vi "Traverse_Space_for new collision code.vi"(9 "Show Panel?":bool, 10 "Traverse Setup":string) -> (3 "Error Comments":string)   [LabVIEW 2016]
doc: "This is an example of using features of the VI Server as a client. It shows how you might browse from one or more applications that may be exporting data from one or more data stations. \n\nThe example shows how to query a server for its list of exported VIs, how to get references to the VIs, and how call them with the Call By Reference function."
uses:
  Route mapping/Box_size.ctl
  Controls/ok_button.ctl
  Collision_Detection/Triangles/EnFlo specific/Collision Detection global.vi
  Globals/Constants_global.vi
  Route mapping/Route_mapping_global.vi
panel:
  in  "Model Name":u16(ring) items=["DIPLOS_array", "Elysee", "Elysee_original", "Elysee_Source1", "Elysee_Source2", "Elysee_Source3", "MAGIC_London_Southbank_0_deg", "MAGIC_London_Southbank_0_deg_excl_12_and_150", "None", "Simple_C", "Simple_V"]
  in  "Traverse Name":u16(ring) items=["EnFlo_Stack", "EnFlo_Trav1", "EnFlo_Trav3", "EnFlo_Trav4", "EnFlo_Tunnel", "EnFlo_Turntable"]
  in  "Cancel Button":bool
  in  "OK":T1
  in  "Traverse Limits":T2=[{"Max"=15001.0, "Min"=12000.0}, {"Max"=1000.0, "Min"=-1000.0}, {"Max"=700.0, "Min"=0.0}] {"Min" format="%#.1f"; "Max" format="%#.1f"}
  # "Enter all coordinates assuming the Model Orientation is zero degrees"
  # "X                           Y                          Z"
  # "All geometry always reloaded after running this panel"
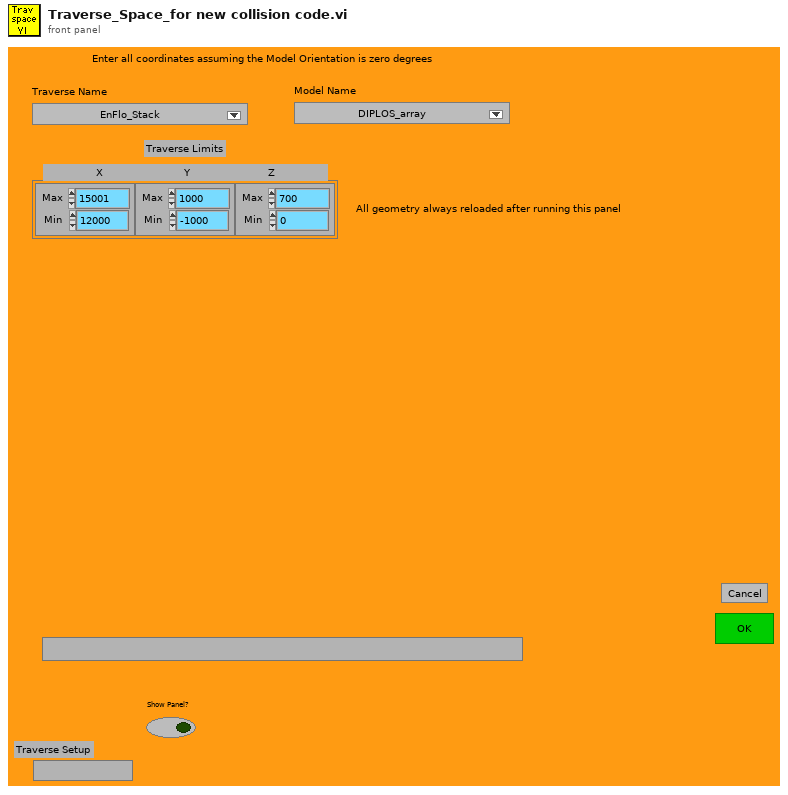
[diagram p1: front panel]
types:
  T1 = typedef "ok_button.ctl" = bool
  T2 = typedef "Box_size.ctl" = cluster{"Max":sgl, "Min":sgl}[]
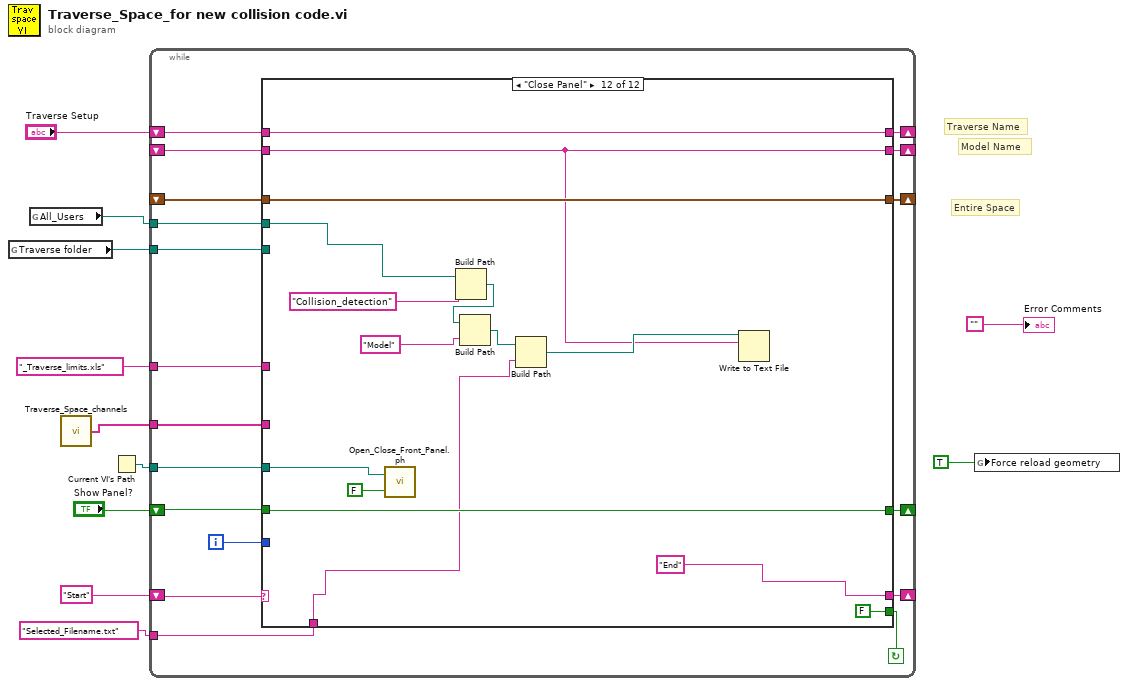
[diagram p0: block diagram]
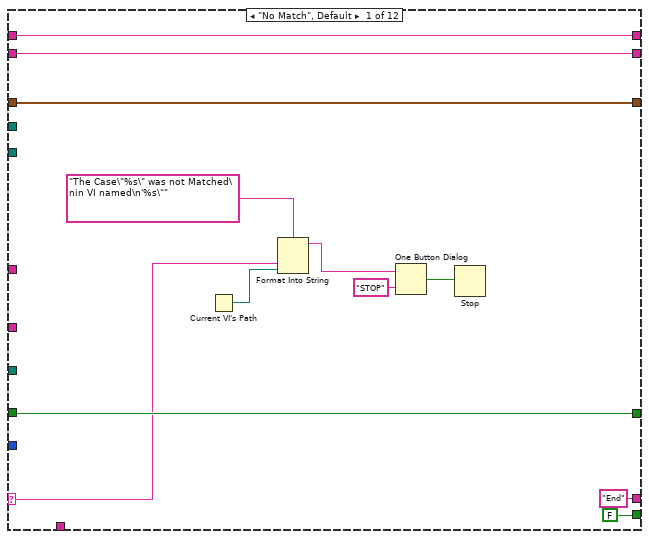
[diagram p2: hidden frame]
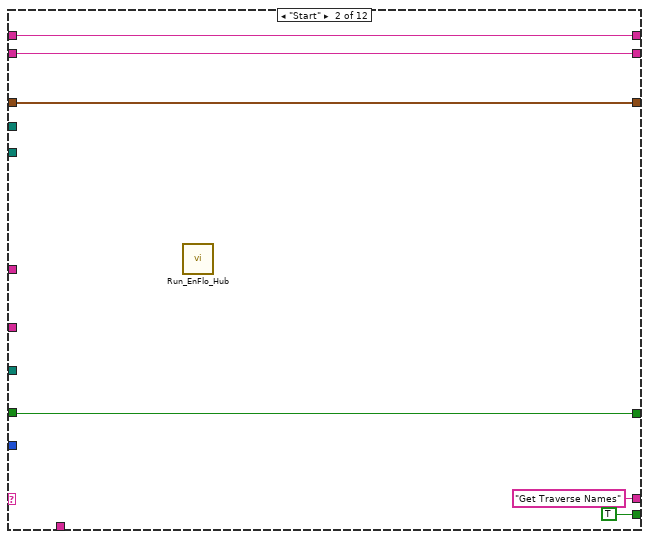
[diagram p3: hidden frame]
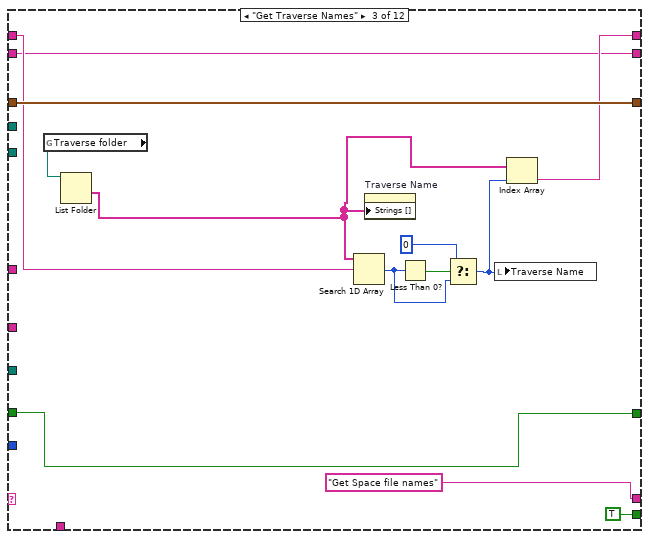
[diagram p4: hidden frame]
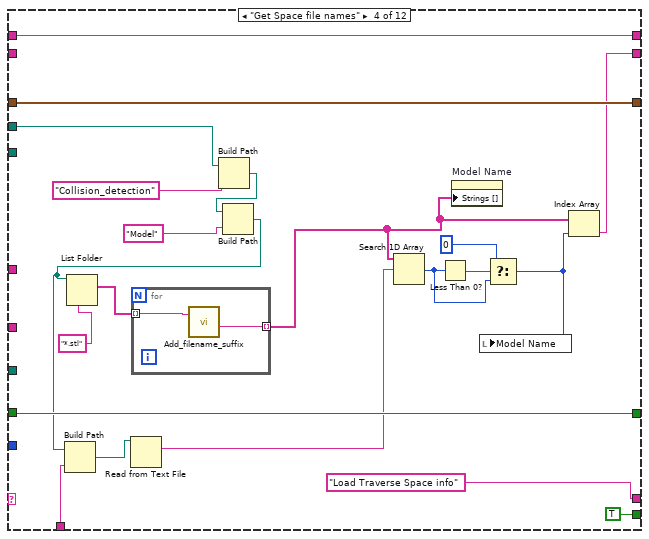
[diagram p5: hidden frame]
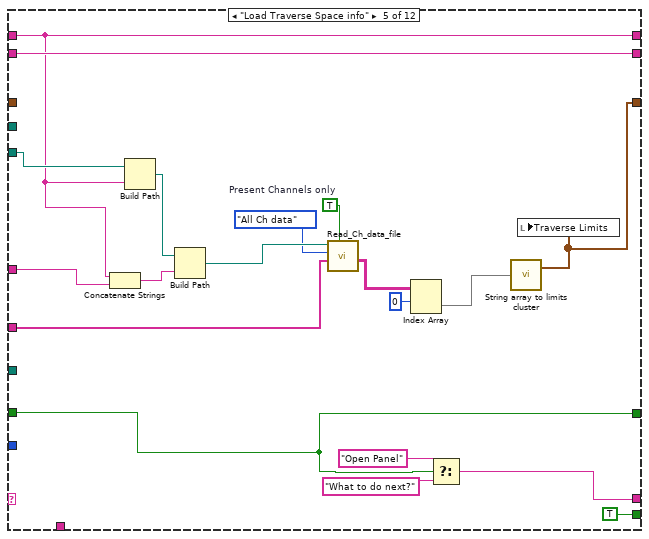
[diagram p6: hidden frame]
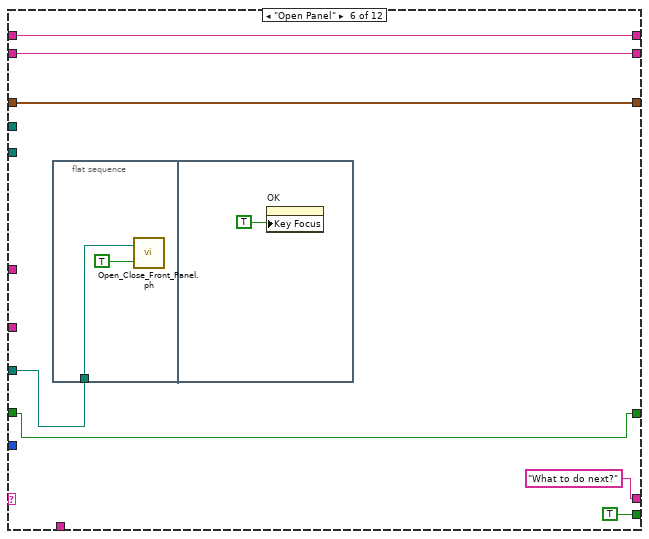
[diagram p7: hidden frame]
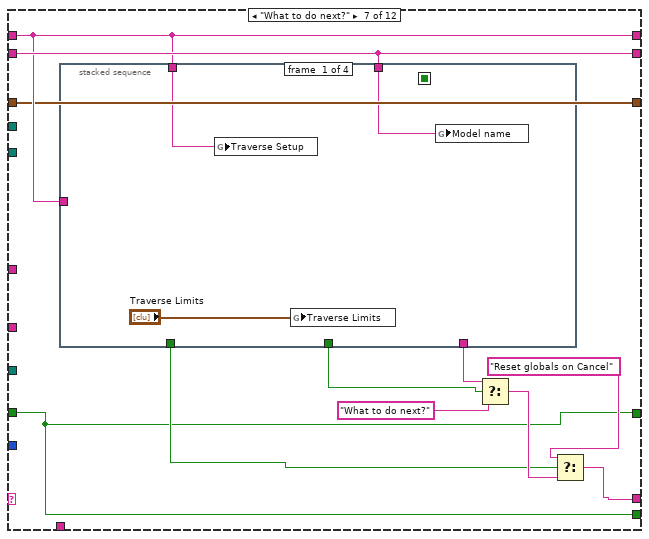
[diagram p8: hidden frame]
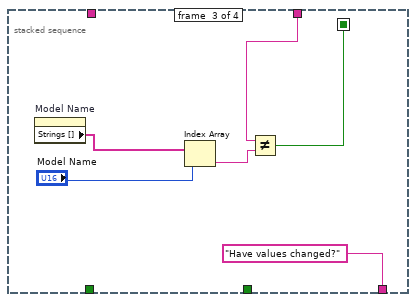
[diagram p10: hidden frame]
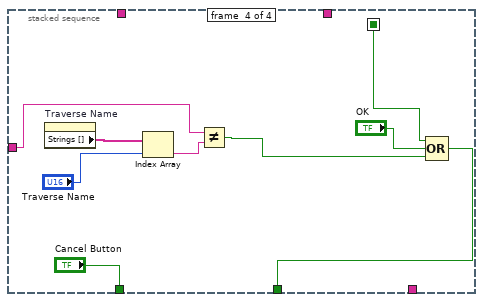
[diagram p11: hidden frame]
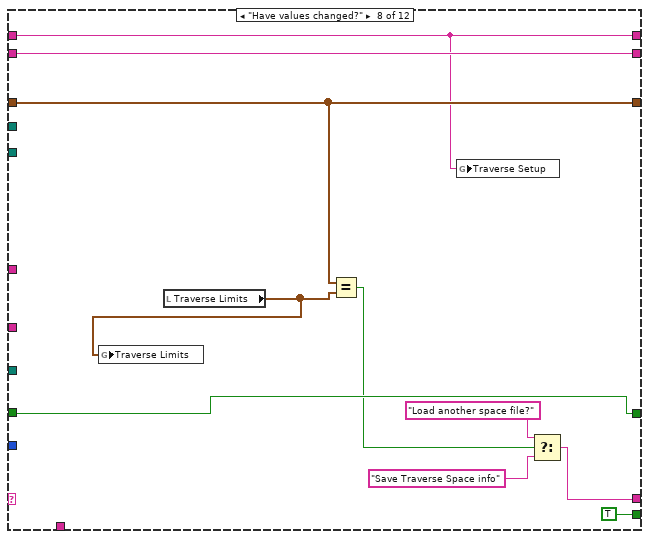
[diagram p12: hidden frame]
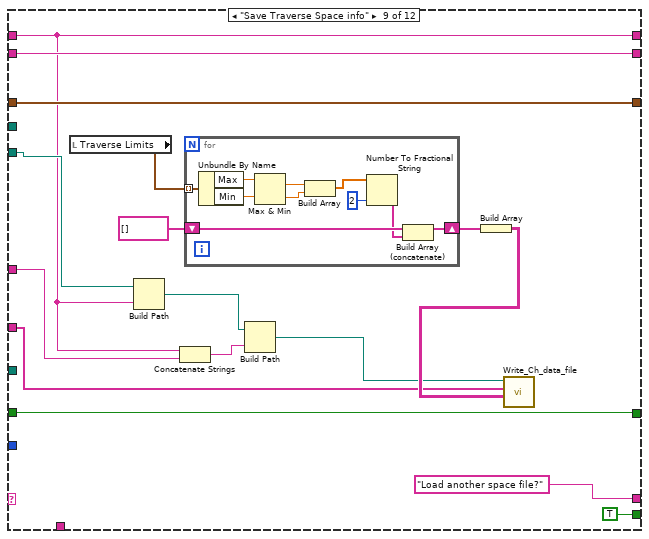
[diagram p13: hidden frame]
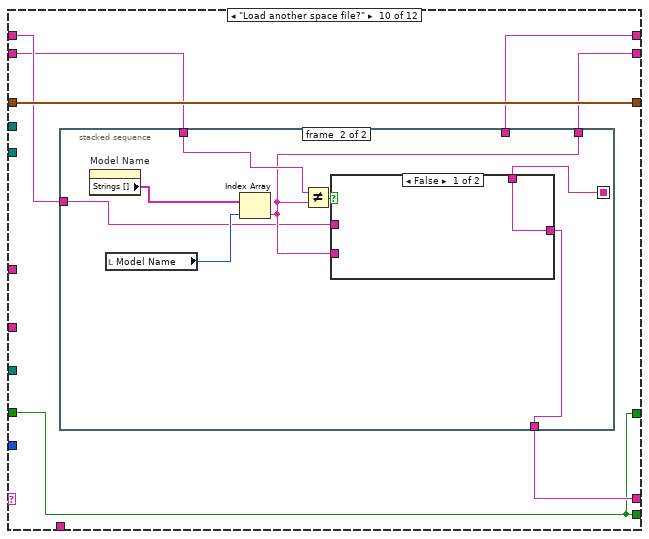
[diagram p14: hidden frame]
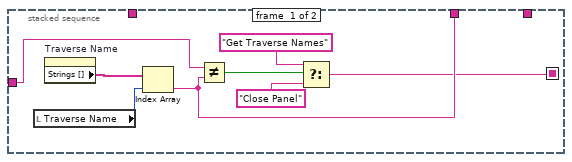
[diagram p15: hidden frame]
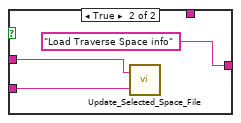
[diagram p16: hidden frame]
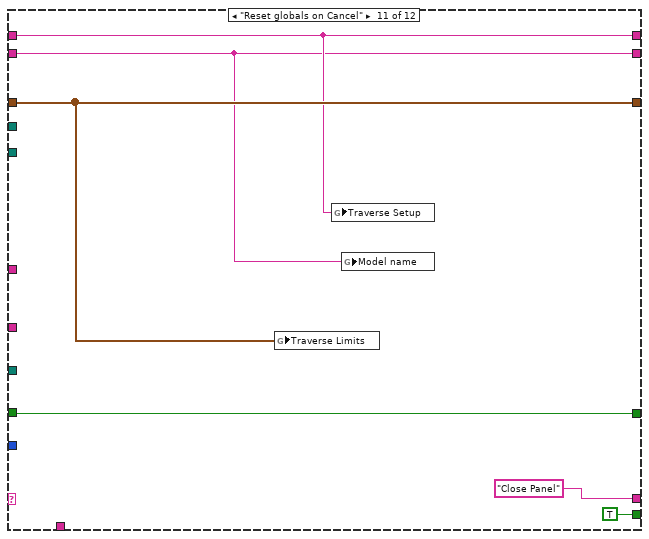
[diagram p17: hidden frame]
diagram:
  # "Traverse Name"
  # "Model Name"
  # "Entire Space"
  n1 = global read "Constants_global.vi" "Traverse folder"() -> (w7:path)
  n2 = global read "Constants_global.vi" "All_Users"() -> (w4:path)
  n3 = call "Traverse_Space_channels.vi"() -> ("Channel Names"=w5:string[])
  n4 = Current VI's Path() -> (path=w10:path)
  n5 = while {
    shift-left: "Start" -> [w25]
    shift-right: [w27] -> _
    tunnel: w10 -> [w26]
    shift-right: [w24] -> _
    shift-left: _ -> [w23]
    shift-right: [w21] -> _
    shift-left: "Traverse Setup" -> [w19]
    shift-right: [w22] -> _
    shift-left: _ -> [w20]
    shift-right: [w17] -> _
    shift-left: "Show Panel?" -> [w18]
    tunnel: w7 -> [w16]
    tunnel: "_Traverse_limits.xls" ("string") -> [w15]
    tunnel: w5 -> [w14]
    tunnel: w4 -> [w13]
    tunnel: "Selected_Filename.txt" ("Substring") -> [w12]
    i -> [w29]
    stop <- w28 continue-if-true
    n6 = case shown="\"Close Panel\"" w25 {
      tunnel: w29 -> [_ _ _ _ _ _ _ _ _ _ _ _]
      tunnel: [FALSE ("status") TRUE ("status") TRUE ("status") TRUE ("status") TRUE ("status") TRUE ("status") w114 TRUE ("status") TRUE ("status") w178 TRUE ("status") FALSE ("status")] -> w28
      selector: w25 -> [w30 _ _ _ _ _ _ _ _ _ _ _]
      tunnel: ["End" ("f") "Get Traverse Names" ("f") "Get Space file names" "Load Traverse Space info" w101 "What to do next?" w122 w147 "Load another space file?" w179 "Close Panel" "End"] -> w27
      tunnel: w18 -> [w31 w42 w49 w71 w87 w103 w114 w145 w163 w178 w207 w218]
      tunnel: w26 -> [_ _ _ _ _ w106 _ _ _ _ _ w222]
      tunnel: [w34 w47 w58 w79 w90 w107 w113 w151 w165 w184 w209 w221] -> w24
      tunnel: w23 -> [w34 w47 w58 w79 _ w107 w113 w151 w165 w184 w209 w221]
      tunnel: [w32 w43 w48 w73 w98 w104 w118 w146 w164 w180 w205 w211] -> w22
      tunnel: [w33 w44 w51 w72 w85 w105 w115 w143 w153 w182 w206 w220] -> w21
      tunnel: w20 -> [w32 w43 w48 _ w98 w104 w118 w146 w164 w181 w205 w211]
      tunnel: w19 -> [w33 w44 w53 w72 w85 w105 w115 w143 w153 w183 w206 w220]
      tunnel: [w31 w42 w49 w71 w87 w103 w114 w145 w163 w178 w207 w218] -> w17
      tunnel: w16 -> [_ _ _ _ w86 _ _ _ w154 _ _ _]
      tunnel: w15 -> [_ _ _ _ w89 _ _ _ w156 _ _ _]
      tunnel: w14 -> [_ _ _ _ w88 _ _ _ w155 _ _ _]
      tunnel: w13 -> [_ _ _ w64 _ _ _ _ _ _ _ w213]
      tunnel: w12 -> [_ _ _ w63 _ _ _ _ _ _ _ w212]
      frame "No Match", Default {
        n7 = Current VI's Path() -> (path=w41:path)
        n8 = Format Into String(format string="The Case\"%s\" was not Matched\nin VI named\n'%s\"" ("Format String"), w30, w41) -> (resulting string=w38:string)  [unwired: 2 in, 1 out]
        n9 = One Button Dialog(message=w38, button name ("OK")="STOP") -> (true=w40:bool)
        n10 = Stop(stop? (T)=w40) -> ()
      }
      frame "Start" {
        n11 = call "Run_EnFlo_Hub.vi"() -> ()  [unwired: 1 in, 7 out]
      }
      frame "Get Traverse Names" {
        n12 = global read "Constants_global.vi" "Traverse folder"() -> (w52:path)
        n13 = List Folder(path=w52) -> (folder names=w50:string[])  [unwired: 1 in, 5 out]
        n14 = Search 1D Array(1D array=w50, element=w53) -> (index of element=w56:i32)  [unwired: 1 out]
        n15 = property on="Traverse Name" class="Ring (strict)"("Strings []"=w50) -> ()  [unwired: 2 in, 2 out]
        n16 = Less Than 0?(x=w56) -> (x < 0?=w57:bool)
        n17 = Select(t=0, s=w57, f=w56) -> (s? t:f=w54:i32)
        n18 = local write "Traverse Name"(w54) -> ()
        n19 = Index Array(array=w50, index=w54) -> (element=w51:string)
      }
      frame "Get Space file names" {
        n20 = Build Path(base path=w64, name or relative path="Collision_detection" ("Substring")) -> (appended path=w70:path)
        n21 = Build Path(base path=w70, name or relative path="Model" ("Substring")) -> (appended path=w67:path)
        n22 = Build Path(base path=w67, name or relative path=w63) -> (appended path=w66:path)
        n23 = List Folder(path=w67, pattern="*.stl") -> (filenames=w62:string[])  [unwired: 1 in, 4 out]
        n24 = Read from Text File(file (use dialog)=w66) -> (text=w65:string)  [unwired: 3 in, 3 out]
        n25 = for {
          tunnel: w62 -> [w83] mode=indexing
          tunnel: [w82] -> w61 mode=indexing
          n26 = call "Add_filename_suffix.vi"("Filename"=w83) -> ("Base name"=w82:string)  [unwired: 1 in, 3 out]
        }
        n27 = Search 1D Array(1D array=w61, element=w65) -> (index of element=w77:i32)  [unwired: 1 out]
        n28 = Less Than 0?(x=w77) -> (x < 0?=w78:bool)
        n29 = property on="Model Name" class="Ring (strict)"("Strings []"=w61) -> ()  [unwired: 2 in, 2 out]
        n30 = Select(t=0, s=w78, f=w77) -> (s? t:f=w74:i32)
        n31 = local write "Model Name"(w74) -> ()
        n32 = Index Array(array=w61, index=w74) -> (element=w73:string)
      }
      frame "Load Traverse Space info" {
        w92 = TRUE  # Present Channels only
        n33 = Concatenate Strings(w85, w89) -> (w93:string)
        n34 = Build Path(base path=w86, name or relative path=w85) -> (appended path=w84:path)
        n35 = Build Path(base path=w84, name or relative path=w93) -> (appended path=w94:path)
        n36 = call "Read_Ch_data_file.vi"("Present Channels only"=w92, "Present Channels"=w88, "Output"=enum16{"All Ch data", "The last few rows"}."All Ch data", "Filename"=w94) -> ("Channel Values"=w95:string[][])  [unwired: 1 in, 4 out]
        n37 = Index Array(array=w95, index (row)=0) -> (element=w97:string[])  [unwired: 1 in]
        n38 = Select(t="Open Panel", s=w87, f="What to do next?") -> (s? t:f=w101:string)
        n39 = call "String array to limits cluster.vi"("Channel Values in"=w97) -> ("Limits out"=w90:T2)  [unwired: 1 out]
        n40 = local write "Traverse Limits"(w90) -> ()
      }
      frame "Open Panel" {
        n41 = flat-sequence {
          tunnel: w106 -> [w110]
          frame #0 {
            n42 = call "Open_Close_Front_Panel.ph.vi"("Front Panel Window:Open"=TRUE, "VI path"=w110) -> ()  [unwired: 2 out]
          }
          frame #1 {
            n43 = property on="OK" class="Bool"("Key Focus"=TRUE) -> ()  [unwired: 2 in, 2 out]
          }
        }
      }
      frame "What to do next?" {
        n44 = stacked-sequence {
          seq-local: [_ _ w128 _] -> [_ _ _ w133]
          tunnel: w115 -> [_ _ _ w138]
          tunnel: [_ _ _ w134] -> w120
          tunnel: [_ _ _ "Cancel Button"] -> w119
          tunnel: w118 -> [w125 _ w129 _]
          tunnel: [_ _ "Have values changed?" _] -> w116
          tunnel: w115 -> [w126 _ _ _]
          frame #0 {
            n45 = global write "Route_mapping_global.vi" "Traverse Setup"(w126) -> ()
            n46 = global write "Route_mapping_global.vi" "Traverse Limits"("Traverse Limits") -> ()
            n47 = global write "Collision Detection global.vi" "Model name"(w125) -> ()
          }
          frame #1 {
            # "Show model pictures here!!"
          }
          frame #2 {
            n48 = property on="Model Name" class="Ring (strict)"() -> ("Strings []"=w131:string[])  [unwired: 2 in, 2 out]
            n49 = Index Array(array=w131, index="Model Name") -> (element=w132:string)
            n50 = Not Equal?(x=w129, y=w132) -> (x != y?=w128:bool)
          }
          frame #3 {
            n51 = property on="Traverse Name" class="Ring (strict)"() -> ("Strings []"=w139:string[])  [unwired: 2 in, 2 out]
            n52 = Index Array(array=w139, index="Traverse Name") -> (element=w137:string)
            n53 = Not Equal?(x=w138, y=w137) -> (x != y?=w136:bool)
            n54 = Compound Arithmetic op=OR(w133, "OK", w136) -> (w134:T1)
          }
        }
        n55 = Select(t=w116, s=w120, f="What to do next?") -> (s? t:f=w123:string)
        n56 = Select(t="Reset globals on Cancel", s=w119, f=w123) -> (s? t:f=w122:string)
      }
      frame "Have values changed?" {
        n57 = local read "Traverse Limits"() -> (w144:T2)
        n58 = global write "Route_mapping_global.vi" "Traverse Limits"(w144) -> ()
        n59 = Equal?(x=w151, y=w144) -> (x = y?=w142:bool)
        n60 = global write "Route_mapping_global.vi" "Traverse Setup"(w143) -> ()
        n61 = Select(t="Load another space file?", s=w142, f="Save Traverse Space info") -> (s? t:f=w147:string)
      }
      frame "Save Traverse Space info" {
        n62 = local read "Traverse Limits"() -> (w157:T2)
        n63 = Build Path(base path=w154, name or relative path=w153) -> (appended path=w152:path)
        n64 = Concatenate Strings(w153, w156) -> (w159:string)
        n65 = for {
          shift-right: [w173] -> w161
          shift-left: string[] [] -> [w175]
          tunnel: w157 -> [w170] mode=indexing
          n66 = Unbundle By Name(w170) -> ("Max"=w169:sgl, "Min"=w168:sgl)
          n67 = Max & Min(x=w169, y=w168) -> (max(x,y)=w172:sgl, min(x,y)=w171:sgl)
          n68 = Build Array(w172, w171) -> (w177:sgl[])
          n69 = Number To Fractional String(number=w177, precision (6)=i16 2) -> (F-format string=w174:string[])  [unwired: 2 out]
          n70 = Build Array (concatenate)(w175, w174) -> (w173:string[])
        }
        n71 = Build Path(base path=w152, name or relative path=w159) -> (appended path=w160:path)
        n72 = Build Array(w161) -> (w162:string[][])
        n73 = call "Write_Ch_data_file.vi"("Channel Values"=w162, "Channel names"=w155, "Filename"=w160) -> ()  [unwired: 4 in, 5 out]
      }
      frame "Load another space file?" {
        n74 = stacked-sequence {
          seq-local: [w186 _] -> [_ w195]
          tunnel: w183 -> [w191 w193]
          tunnel: [w187 _] -> w182
          tunnel: [_ w198] -> w179
          tunnel: w181 -> [_ w197]
          tunnel: [_ w194] -> w180
          frame #0 {
            n75 = local read "Traverse Name"() -> (w185:u16)
            n76 = property on="Traverse Name" class="Ring (strict)"() -> ("Strings []"=w192:string[])  [unwired: 2 in, 2 out]
            n77 = Index Array(array=w192, index=w185) -> (element=w187:string)
            n78 = Not Equal?(x=w191, y=w187) -> (x != y?=w190:bool)
            n79 = Select(t="Get Traverse Names" ("f"), s=w190, f="Close Panel") -> (s? t:f=w186:string)
          }
          frame #1 {
            n80 = property on="Model Name" class="Ring (strict)"() -> ("Strings []"=w200:string[])  [unwired: 2 in, 2 out]
            n81 = local read "Model Name"() -> (w199:u16)
            n82 = Index Array(array=w200, index=w199) -> (element=w194:string)
            n83 = Not Equal?(x=w197, y=w194) -> (x != y?=w196:bool)
            n84 = case shown="False" w196 {
              tunnel: [w201 "Load Traverse Space info" ("f")] -> w198
              tunnel: w195 -> [w201 _]
              tunnel: w194 -> [_ w203]
              tunnel: w193 -> [_ w202]
              frame False {
              }
              frame True {
                n85 = call "Update_Selected_Space_File.vi"("Selected Space File Name"=w203, "Traverse Setup"=w202) -> ()  [unwired: 1 in]
              }
            }
          }
        }
      }
      frame "Reset globals on Cancel" {
        n86 = global write "Route_mapping_global.vi" "Traverse Limits"(w209) -> ()
        n87 = global write "Route_mapping_global.vi" "Traverse Setup"(w206) -> ()
        n88 = global write "Collision Detection global.vi" "Model name"(w205) -> ()
      }
      frame "Close Panel" {
        n89 = call "Open_Close_Front_Panel.ph.vi"("Front Panel Window:Open"=FALSE, "VI path"=w222) -> ()  [unwired: 2 out]
        n90 = Build Path(base path=w213, name or relative path="Collision_detection" ("Substring")) -> (appended path=w215:path)
        n91 = Build Path(base path=w215, name or relative path="Model" ("Substring")) -> (appended path=w214:path)
        n92 = Build Path(base path=w214, name or relative path=w212) -> (appended path=w219:path)
        n93 = Write to Text File(file (use dialog)=w219, text=w211) -> ()  [unwired: 2 in, 3 out]
      }
    }
  }
  n94 = global write "Collision Detection global.vi" "Force reload geometry"(TRUE ("Reload geometry")) -> ()
  "Error Comments" <- ""
